vi "S2C_InitEvent.vi"(8 "Error In":errorcluster) -> (0 "Error Out":errorcluster)   [LabVIEW 2015]
doc: "Detects an error and calls the error case to process the error."
uses:
  Globals/S2C_Globals.vi
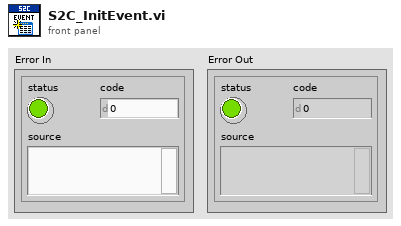
[diagram p1: front panel]
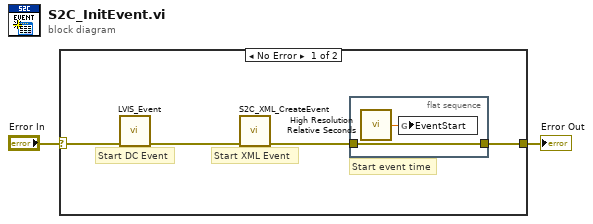
[diagram p0: block diagram]
diagram:
  n1 = case shown="No Error" "Error In" {
    selector: "Error In" -> [w5 w9]
    tunnel: [w3 w9] -> w1
    frame No Error {
      # "Start event time"
      # "Start XML Event"
      # "Start DC Event"
      n2 = call "LVIS_Event.vi"("Error In"=w5) -> ("Error Out"=w6:errorcluster)  [unwired: 10 in]
      n3 = call "S2C_XML_CreateEvent.vi"("Error In"=w6) -> ("Error Out"=w4:errorcluster)  [unwired: 10 in]
      n4 = flat-sequence {
        tunnel: w4 -> [w7]
        tunnel: [w7] -> w3
        frame #0 {
          n5 = call <vilib>:"High Resolution Relative Seconds.vi"() -> ("relative seconds"=w8:dbl)
          n6 = global write "S2C_Globals.vi" "EventStart"(w8) -> ()
        }
      }
    }
    frame Error {
    }
  }
  "Error Out" <- w1
